vi "g_ReportControl.vi"() -> ()   [LabVIEW 2014]
uses:
  c_ReportMessages.ctl
panel:
  out "selected path":path
  in  "Combo Box":T1
  in  "New Report":bool
  in  "Write":bool
  in  "Report Enable":bool
  in  "Report String":string
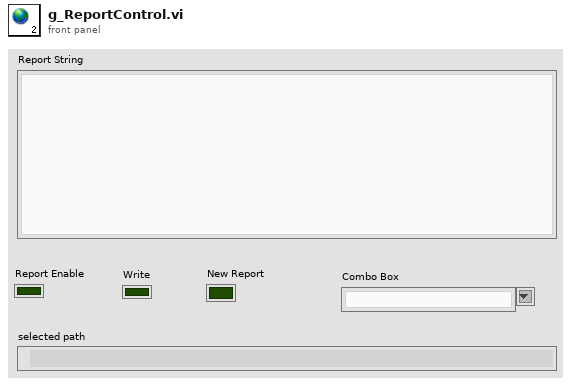
[diagram p1: front panel]
types:
  T1 = typedef "c_ReportMessages.ctl" = string
diagram:
